vi "多通道二维图.vi"() -> ()   [LabVIEW 2023]
uses:
  <vilib>/Utility/file.llb/Read Delimited Spreadsheet (string).vi
panel:
  out "XY Graph":cluster{dbl[], dbl[]}[](graph)
  out "subarray":string[][](array[string])
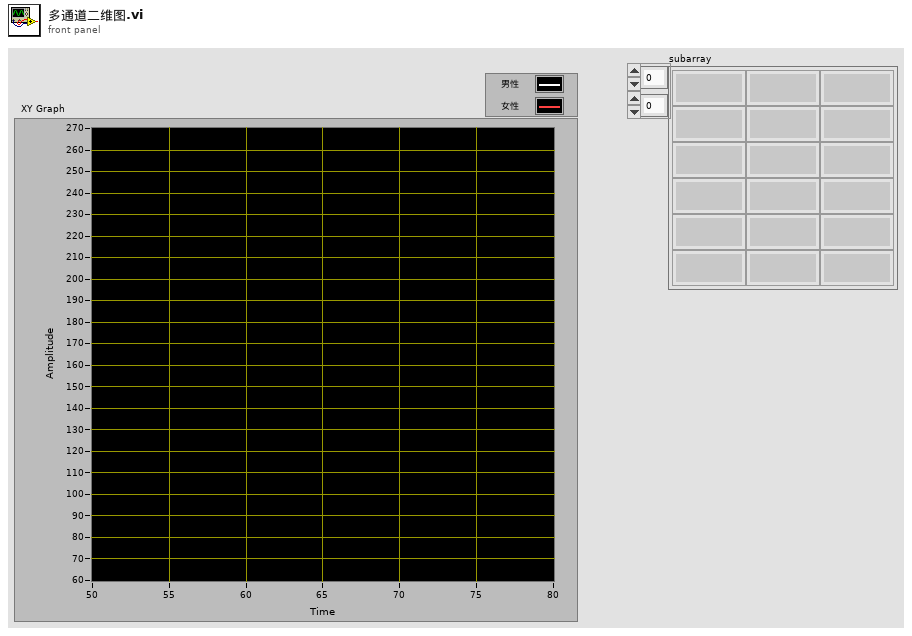
[diagram p1: front panel]
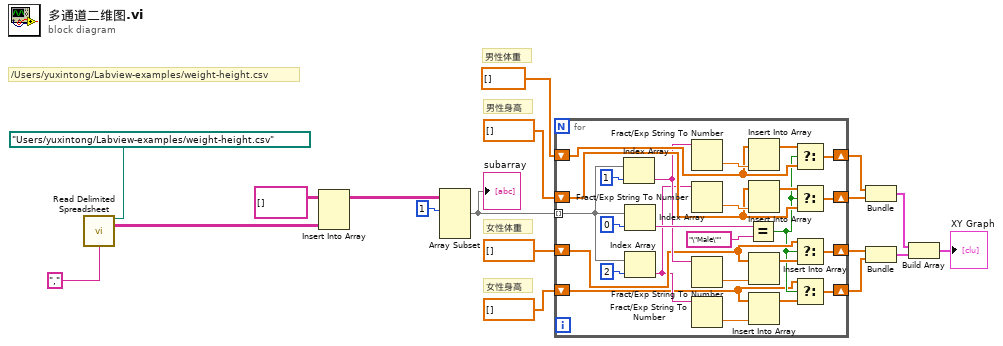
[diagram p0: block diagram]
diagram:
  # "女性身高"
  # "女性体重"
  # "男性身高"
  # "男性体重"
  # "/Users/yuxintong/Labview-examples/weight-height.csv"
  n1 = call-poly <vilib>:"Read Delimited Spreadsheet.vi"("file path (dialog if empty)"=path "/Users/yuxintong/Labview-examples/weight-height.csv", "delimiter (\\t)"="," ("delimiter (\\t)")) -> ("all rows"=w15:string[][])  [unwired: 8 in, 5 out]
  n2 = Insert Into Array "Insert Into Array"(array=string[][] [], new element=w15) -> (w14:string[][])  [unwired: 2 in]
  n3 = Array Subset(array=w14, index (row)=1 ("index")) -> (w12:string[][])  [unwired: 3 in]
  "subarray" <- w12
  n4 = for {
    tunnel: w12 -> [w42] mode=indexing
    shift-right: [w34] -> w5
    shift-left: dbl[] [] -> [w35]
    shift-right: [w30] -> w4
    shift-left: dbl[] [] -> [w31]
    shift-right: [w25] -> w7
    shift-left: dbl[] [] -> [w26]
    shift-right: [w19] -> w6
    shift-left: dbl[] [] -> [w20]
    n5 = Index Array(array=w42, index=1) -> (element=w29:string)
    n6 = Index Array(array=w42, index=0) -> (element=w39:string)
    n7 = Index Array(array=w42, index=2) -> (element=w24:string)
    n8 = Fract/Exp String To Number(string=w29) -> (number=w37:dbl)  [unwired: 3 in, 1 out]
    n9 = Fract/Exp String To Number(string=w24) -> (number=w33:dbl)  [unwired: 3 in, 1 out]
    n10 = Fract/Exp String To Number(string=w29) -> (number=w28:dbl)  [unwired: 3 in, 1 out]
    n11 = Fract/Exp String To Number(string=w24) -> (number=w23:dbl)  [unwired: 3 in, 1 out]
    n12 = Equal?(x=w39, y="\"Male\"") -> (x = y?=w22:bool)
    n13 = Insert Into Array(array=w35, new element=w37) -> (w36:dbl[])  [unwired: 1 in]
    n14 = Insert Into Array(array=w31, new element=w33) -> (w32:dbl[])  [unwired: 1 in]
    n15 = Insert Into Array(array=w26, new element=w28) -> (w27:dbl[])  [unwired: 1 in]
    n16 = Insert Into Array(array=w20, new element=w23) -> (w21:dbl[])  [unwired: 1 in]
    n17 = Select(t=w36, s=w22, f=w35) -> (s? t:f=w34:dbl[])
    n18 = Select(t=w32, s=w22, f=w31) -> (s? t:f=w30:dbl[])
    n19 = Select(t=w26, s=w22, f=w27) -> (s? t:f=w25:dbl[])
    n20 = Select(t=w20, s=w22, f=w21) -> (s? t:f=w19:dbl[])
  }
  n21 = Bundle(w5, w4) -> (w3:cluster{dbl[], dbl[]})  [unwired: 1 in]
  n22 = Bundle(w7, w6) -> (w2:cluster{dbl[], dbl[]})  [unwired: 1 in]
  n23 = Build Array(w3, w2) -> (→"XY Graph":cluster{dbl[], dbl[]}[])
